vi "InitDLLs_old.vi"(0 "scenarios2VirtPlantOutputMsgs":refnum<vi>, 1 "scenarios2VerifierOutputMsgs":refnum<vi>, 2 "algOutputMsgs":refnum<vi>, 3 "verifier2GUIOutputMsgs":refnum<vi>, 4 "virtualPlant2GUIOutputMsgs":refnum<vi>, 5 "algStates":refnum<vi>, 6 "scenarios2AlgOutputMsgs":refnum<vi>, 7 "vplantStates":refnum<vi>, 8 "algOutputPorts":refnum<vi>, 9 "verStates":refnum<vi>, 10 "algInputPorts":refnum<vi>, 11 "scenarioStates":refnum<vi>, 18 "verifier2scenariousControlOutMsgs":refnum<vi>) -> ()   [LabVIEW 2010]
uses:
  DLL-s/MakeFullImmitationStepDLL/Release/MakeFullImmitationStepDLL.dll
panel:
  out "error":u8
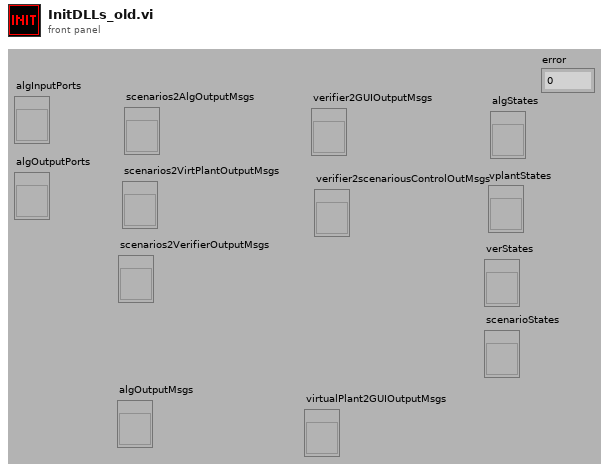
[diagram p1: front panel]
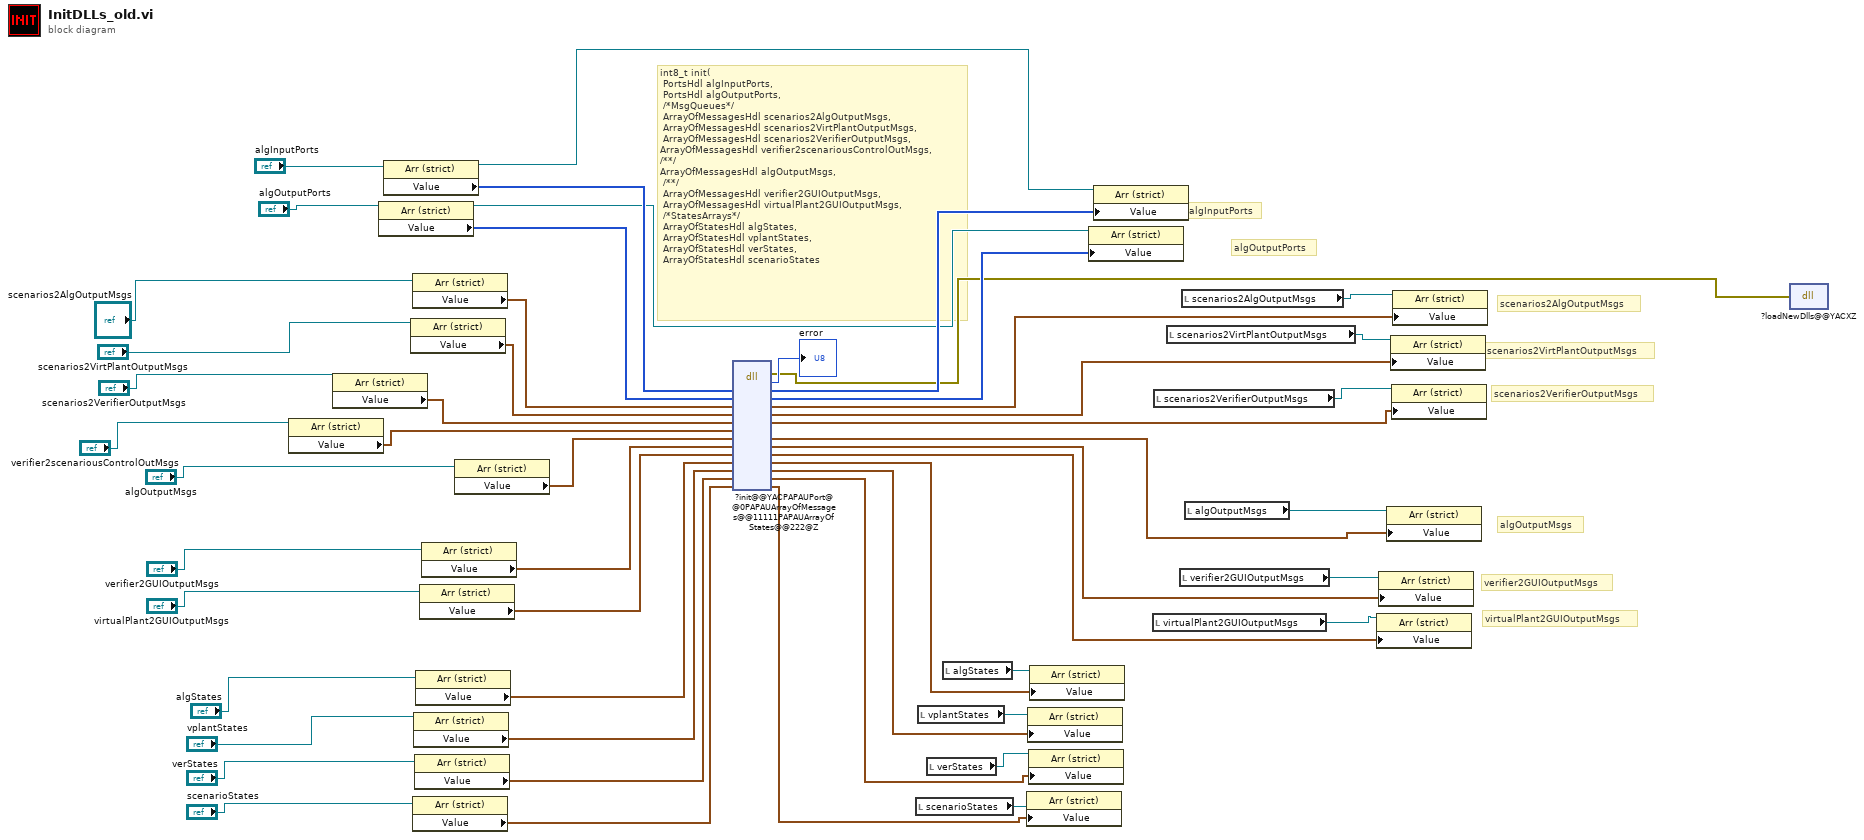
[diagram p0: block diagram]
diagram:
  # "virtualPlant2GUIOutputMsgs"
  # "verifier2GUIOutputMsgs"
  # "algOutputMsgs"
  # "scenarios2VerifierOutputMsgs"
  # "scenarios2VirtPlantOutputMsgs"
  # "scenarios2AlgOutputMsgs"
  # "algOutputPorts"
  # "algInputPorts"
  # "int8_t init(\n\tPortsHdl algInputPorts,\n\tPortsHdl algOutputPorts,\n\t/*MsgQueues*/\n\tArrayOfMessagesHdl scenarios2AlgOutputMsgs,\n\tArrayOfMessagesHdl scenarios2VirtPlantOutputMsgs,\n\tArrayOfMessagesHdl scenarios2VerifierOutputMsgs,\nArrayOfMessagesHdl verifier2scenariousControlOutMsgs,\n/**/\t\nArrayOfMessagesHdl algOutputMsgs,\n\t/**/\n\tArrayOfMessagesHdl verifier2GUIOutputMsgs,\n\tArrayOfMessagesHdl virtualPlant2GUIOutputMsgs,\n\t/*StatesArrays*/\n\tArrayOfStatesHdl algStates,\n\tArrayOfStatesHdl vplantStates,\n\tArrayOfStatesHdl verStates,\n\tArrayOfStatesHdl scenarioStates"
  n1 = property class="Arr (strict)"(reference="verifier2scenariousControlOutMsgs") -> ("Value"=w1:cluster{"MSG":i16, "param":i32, "Type":i16}[])  [unwired: 1 in, 2 out]
  n2 = property class="Arr (strict)"(reference="scenarios2VerifierOutputMsgs") -> ("Value"=w42:cluster{"MSG":i16, "param":i32, "Type":i16}[])  [unwired: 1 in, 2 out]
  n3 = property class="Arr (strict)"(reference="algOutputPorts") -> (reference out=w25:refnum<vi>, "Value"=w45:i8[])  [unwired: 1 in, 1 out]
  n4 = property class="Arr (strict)"(reference="algInputPorts") -> (reference out=w26:refnum<vi>, "Value"=w46:i8[])  [unwired: 1 in, 1 out]
  n5 = property class="Arr (strict)"(reference="scenarios2VirtPlantOutputMsgs") -> ("Value"=w43:cluster{"MSG":i16, "param":i32, "Type":i16}[])  [unwired: 1 in, 2 out]
  n6 = property class="Arr (strict)"(reference="scenarios2AlgOutputMsgs") -> ("Value"=w44:cluster{"MSG":i16, "param":i32, "Type":i16}[])  [unwired: 1 in, 2 out]
  n7 = property class="Arr (strict)"(reference="scenarioStates") -> ("Value"=w29:cluster{"TimeInState":u16, "cur_state":i8}[])  [unwired: 1 in, 2 out]
  n8 = property class="Arr (strict)"(reference="vplantStates") -> ("Value"=w31:cluster{"TimeInState":u16, "cur_state":i8}[])  [unwired: 1 in, 2 out]
  n9 = property class="Arr (strict)"(reference="verStates") -> ("Value"=w30:cluster{"TimeInState":u16, "cur_state":i8}[])  [unwired: 1 in, 2 out]
  n10 = property class="Arr (strict)"(reference="algStates") -> ("Value"=w32:cluster{"TimeInState":u16, "cur_state":i8}[])  [unwired: 1 in, 2 out]
  n11 = property class="Arr (strict)"(reference="virtualPlant2GUIOutputMsgs") -> ("Value"=w37:cluster{"MSG":i16, "param":i32, "Type":i16}[])  [unwired: 1 in, 2 out]
  n12 = property class="Arr (strict)"(reference="verifier2GUIOutputMsgs") -> ("Value"=w38:cluster{"MSG":i16, "param":i32, "Type":i16}[])  [unwired: 1 in, 2 out]
  n13 = property class="Arr (strict)"(reference="algOutputMsgs") -> ("Value"=w41:cluster{"MSG":i16, "param":i32, "Type":i16}[])  [unwired: 1 in, 2 out]
  n14 = dll-call lib="D:/Liakh Tanya/Dissertation/Complex/DLL-s/MakeFullImmitationStepDLL/Release/MakeFullImmitationStepDLL.dll" fn="?init@@YACPAPAUPort@@0PAPAUArrayOfMessages@@11111PAPAUArrayOfStates@@222@Z" label="Init"("algInputPorts"=w46, "algOutputPorts"=w45, "scenarios2AlgOutputMsgs"=w44, "scenarios2VirtPlantOutputMsgs"=w43, "scenarios2VerifierOutputMsgs"=w42, "verifier2scenariousControlOutMsgs,"=w1, "algOutputMsgs"=w41, "verifier2GUIOutputMsgs"=w38, "virtualPlant2GUIOutputMsgs"=w37, "algStates"=w32, "vplantStates"=w31, "verStates"=w30, "scenarioStates"=w29) -> (error out=w3:errorcluster, "error"=→"error":i8, "algInputPorts"=w28:i8[], "algOutputPorts"=w27:i8[], "scenarios2AlgOutputMsgs"=w14:cluster{"MSG":i16, "param":i32, "Type":i16}[], "scenarios2VirtPlantOutputMsgs"=w13:cluster{"MSG":i16, "param":i32, "Type":i16}[], "scenarios2VerifierOutputMsgs"=w12:cluster{"MSG":i16, "param":i32, "Type":i16}[], "algOutputMsgs"=w11:cluster{"MSG":i16, "param":i32, "Type":i16}[], "verifier2GUIOutputMsgs"=w10:cluster{"MSG":i16, "param":i32, "Type":i16}[], "virtualPlant2GUIOutputMsgs"=w9:cluster{"MSG":i16, "param":i32, "Type":i16}[], "algStates"=w8:cluster{"TimeInState":u16, "cur_state":i8}[], "vplantStates"=w6:cluster{"TimeInState":u16, "cur_state":i8}[], "verStates"=w5:cluster{"TimeInState":u16, "cur_state":i8}[], "scenarioStates"=w7:cluster{"TimeInState":u16, "cur_state":i8}[])  [unwired: 4 in, 1 out]
  n15 = local read "scenarioStates"() -> (w15:refnum<vi>)
  n16 = local read "vplantStates"() -> (w17:refnum<vi>)
  n17 = local read "verStates"() -> (w16:refnum<vi>)
  n18 = local read "algStates"() -> (w18:refnum<vi>)
  n19 = property class="Arr (strict)"(reference=w15, "Value"=w7) -> ()  [unwired: 1 in, 2 out]
  n20 = property class="Arr (strict)"(reference=w17, "Value"=w6) -> ()  [unwired: 1 in, 2 out]
  n21 = property class="Arr (strict)"(reference=w16, "Value"=w5) -> ()  [unwired: 1 in, 2 out]
  n22 = property class="Arr (strict)"(reference=w18, "Value"=w8) -> ()  [unwired: 1 in, 2 out]
  n23 = property class="Arr (strict)"(reference=w25, "Value"=w27) -> ()  [unwired: 1 in, 2 out]
  n24 = property class="Arr (strict)"(reference=w26, "Value"=w28) -> ()  [unwired: 1 in, 2 out]
  n25 = local read "virtualPlant2GUIOutputMsgs"() -> (w19:refnum<vi>)
  n26 = local read "scenarios2VerifierOutputMsgs"() -> (w22:refnum<vi>)
  n27 = local read "scenarios2VirtPlantOutputMsgs"() -> (w23:refnum<vi>)
  n28 = local read "verifier2GUIOutputMsgs"() -> (w20:refnum<vi>)
  n29 = local read "scenarios2AlgOutputMsgs"() -> (w24:refnum<vi>)
  n30 = local read "algOutputMsgs"() -> (w21:refnum<vi>)
  n31 = property class="Arr (strict)"(reference=w19, "Value"=w9) -> ()  [unwired: 1 in, 2 out]
  n32 = property class="Arr (strict)"(reference=w20, "Value"=w10) -> ()  [unwired: 1 in, 2 out]
  n33 = property class="Arr (strict)"(reference=w21, "Value"=w11) -> ()  [unwired: 1 in, 2 out]
  n34 = property class="Arr (strict)"(reference=w23, "Value"=w13) -> ()  [unwired: 1 in, 2 out]
  n35 = property class="Arr (strict)"(reference=w22, "Value"=w12) -> ()  [unwired: 1 in, 2 out]
  n36 = property class="Arr (strict)"(reference=w24, "Value"=w14) -> ()  [unwired: 1 in, 2 out]
  n37 = dll-call lib="D:/Liakh Tanya/Dissertation/Complex/DLL-s/MakeFullImmitationStepDLL/Release/MakeFullImmitationStepDLL.dll" fn="?loadNewDlls@@YACXZ" label="Load NEW DLLs"(error in=w3) -> ()  [unwired: 3 in, 2 out]
